vi "Move to Zero Position.vi"(0 "reference in":refnum<class "SmartMotor.lvclass">, 5 "error in (no error)":errorcluster) -> (14 "reference out":refnum<class "SmartMotor.lvclass">, 19 "error out":errorcluster)   [LabVIEW 2017, in "SmartMotor.lvclass"]
uses:
  SmartMotor.lvclass
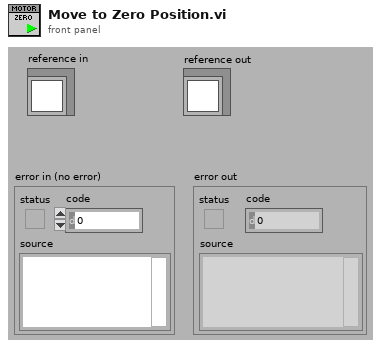
[diagram p1: front panel]
types:
  T1 = typedef "SmartMotor.lvclass/ObjectAttributes.ctl" = cluster{"SmartMotor Chain VISA Resource":refnum<visa-resource-name>, "SmartMotor Chain Address":i16, "Motor Absolute Position":i32, "Motor Relative Position":i32, "Motor Torque":i32, "Motor Voltage":i32, "Screwdriver Engaged":bool, "Screwdriver Torque Limit":i32, "Torque Monitor On/Off Status":bool, "Torque Monitor VI Reference":refnum<vi>, "Absolute Motor Torque (Filtered)":dbl, "SmartMotor Status":T2, "SmartMotor Error":T3}
  T2 = typedef "SmartMotor.lvclass/SmartMotor Status.ctl" = enum8{"Stopped", "Moving"}
  T3 = typedef "SmartMotor.lvclass/SmartMotor Error.ctl" = enum8{"None", "Read Error", "Low Voltage"}
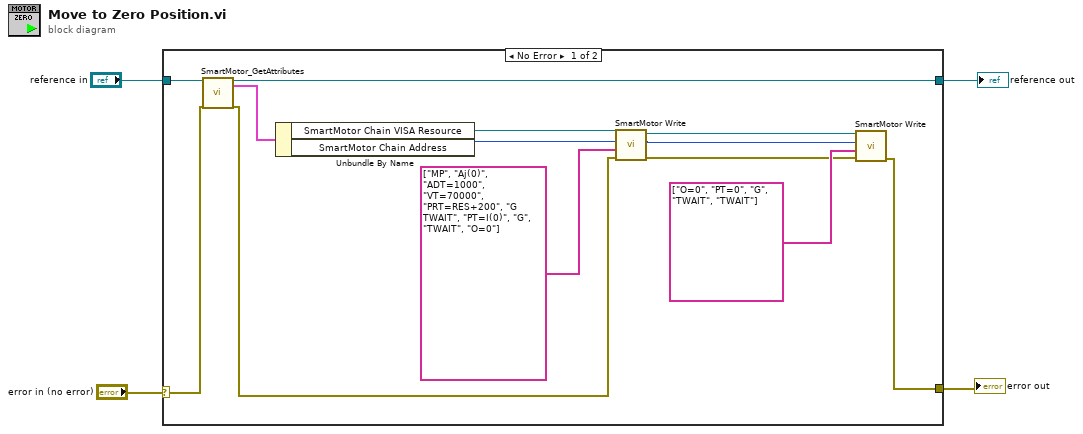
[diagram p0: block diagram]
diagram:
  n1 = case shown="No Error" "error in (no error)" {
    selector: "error in (no error)" -> [w17 w19]
    tunnel: [w8 w19] -> w3
    tunnel: [w14 w18] -> w1
    tunnel: "reference in" -> [w15 w18]
    frame No Error {
      n2 = call "SmartMotor_GetAttributes.vi"("reference in"=w15, "error in (no error)"=w17) -> ("reference out"=w14:refnum<class "SmartMotor.lvclass">, "Data"=w16:T1, "error out"=w7:errorcluster)  [unwired: 14 in, 1 out]
      n3 = Unbundle By Name(w16) -> ("SmartMotor Chain VISA Resource"=w11:refnum<visa-resource-name>, "SmartMotor Chain Address"=w6:i16)
      n4 = call "SmartMotor Write.vi"("VISA resource IN"=w11, "Motor Number"=w6, "Motor Command Array"=string[] ["MP", "Aj(0)", "ADT=1000", "VT=70000", "PRT=RES+200", "G TWAIT", "PT=I(0)", "G", "TWAIT", "O=0"], "Error In"=w7) -> ("VISA resource OUT"=w10:refnum<visa-resource-name>, "Motor Number OUT"=w5:i16, "Error Out"=w9:errorcluster)  [unwired: 3 in]
      n5 = call "SmartMotor Write.vi"("VISA resource IN"=w10, "Motor Number"=w5, "Motor Command Array"=string[] ["O=0", "PT=0", "G", "TWAIT", "TWAIT"], "Error In"=w9) -> ("Error Out"=w8:errorcluster)  [unwired: 3 in, 2 out]
    }
    frame Error {
    }
  }
  "error out" <- w3
  "reference out" <- w1
